vi "Sort Component Subtype.vi"(1 "Array In":T1[](array[typedef])) -> (0 "Array Out":T1[](array[typedef]))   [LabVIEW 2013]
uses:
  Controls/Display Component Line.ctl
  Controls/Components.ctl
  Controls/Component Sub Type.ctl
  Controls/Add Button.ctl
  Controls/Subtract Button.ctl
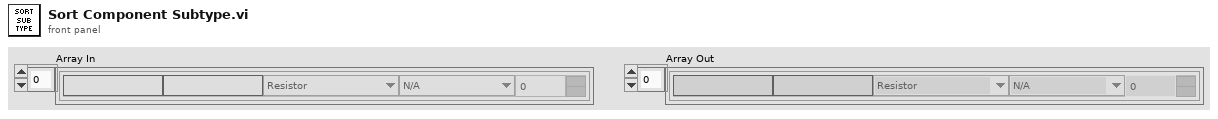
[diagram p1: front panel]
types:
  T1 = typedef "Display Component Line.ctl" = cluster{"Part Number":string, "Code (Value)":string, "Component Type":T2, "Component Subtype":T3, "Quantity":u32, "Add":T4, "Subtract":T5}
  T2 = typedef "Components.ctl" = enum16{"Resistor", "Capacitor", "Diode", "Voltage Regulator", "Transistors", "ICs"}
  T3 = typedef "Component Sub Type.ctl" = enum16{"N/A", "Carbon", "Variable - Trimmer", "Variable - Pot", "Ceramic", "Electrolitic", "Zenner", "TO-92", "TO-220", "NPN", "PNP", "CMOS", "Processor"}
  T4 = typedef "Add Button.ctl" = bool
  T5 = typedef "Subtract Button.ctl" = bool
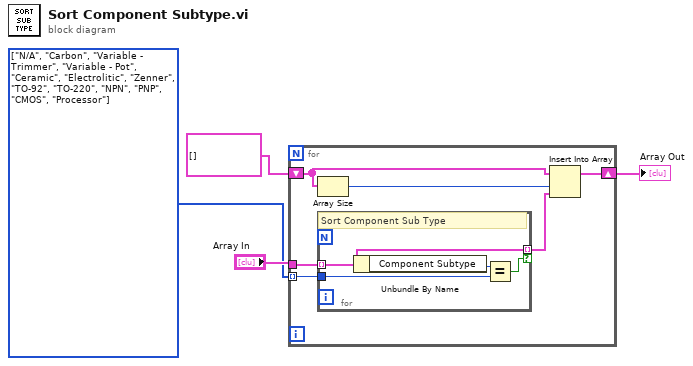
[diagram p0: block diagram]
diagram:
  w1 = T3[] [enum."N/A", enum."Carbon", enum."Variable - Trimmer", enum."Variable - Pot", enum."Ceramic", enum."Electrolitic", enum."Zenner", enum."TO-92", enum."TO-220", enum."NPN", enum."PNP", enum."CMOS", enum."Processor"] items=["N/A", "Carbon", "Variable - Trimmer", "Variable - Pot", "Ceramic", "Electrolitic", "Zenner", "TO-92", "TO-220", "NPN", "PNP", "CMOS", "Processor"]
  n1 = for {
    tunnel: "Array In" -> [w10]
    tunnel: w1 -> [w9] mode=indexing
    shift-right: [w5] -> w4
    shift-left: T1[] [] -> [w8]
    n2 = Array Size(array=w8) -> (size(s)=w7:i32)
    n3 = for {
      tunnel: w10 -> [w12] mode=indexing
      tunnel: w9 -> [w13]
      tunnel: [w12] -> w6 mode=indexing if=w11
      # "Sort Component Sub Type"
      n4 = Unbundle By Name(w12) -> ("Component Subtype"=w14:T3)
      n5 = Equal?(x=w14, y=w13) -> (x = y?=w11:bool)
    }
    n6 = Insert Into Array(array=w8, index=w7, new element=w6) -> (w5:T1[])
  }
  "Array Out" <- w4
